vi "HandleFeedForward.vi"(8 "timed out":bool, 11 "Value":u64) -> ()   [LabVIEW 2018]
uses:
  <vilib>/rvi/Memory/Memory_Emulation/nirvimemoryFastEmulation.vi
  <vilib>/rvi/Memory/Memory_Emulation/nirvimemoryEmulation.vi
  <vilib>/rvi/Emulation/niFpgaEmulationIsFPGAContextNoSignature.vi
  <vilib>/rvi/DataTransferAndStorage/Container/Common/niFpgaContainerGetUniqueNameForEmu.vi
  <vilib>/rvi/Emulation/niFpgaProcessEmulError.vi
  <vilib>/rvi/Emulation/niFpgaSctlEmulationGetInTimedLoop.vi
  <vilib>/rvi/errors/nirviReportUnexpectedCaseInternalError (U32).vi
  <vilib>/rvi/FXPMathLib/FxpInterpret/XNode/nifxpmath_Interpret.xnode
  <vilib>/rvi/DataTransferAndStorage/Container/XNode/niFpgaContainer.xnode
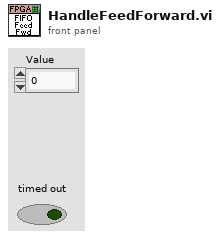
[diagram p1: front panel]
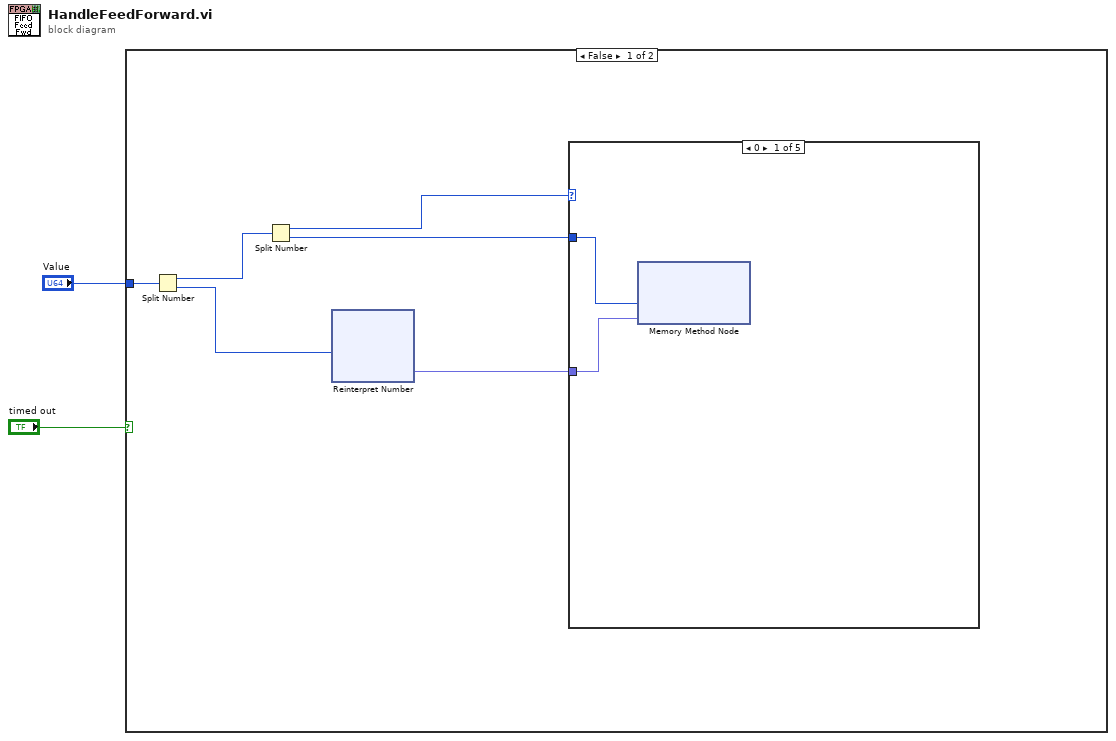
[diagram p0: block diagram]
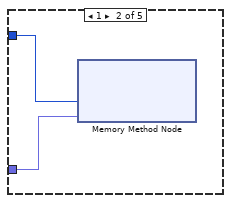
[diagram p2: hidden frame]
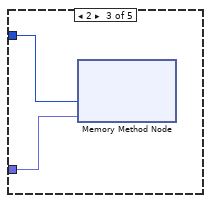
[diagram p3: hidden frame]
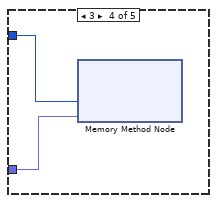
[diagram p4: hidden frame]
diagram:
  n1 = case shown="False" "timed out" {
    tunnel: "Value" -> [w8 _]
    frame False {
      n2 = Split Number(x=w8) -> (hi(x)=w5:u32, lo(x)=w6:u32)
      n3 = Split Number(x=w5) -> (hi(x)=w4:u16, lo(x)=w3:u16)
      n4 = xnode "Reinterpret Number"("x"=w6) -> ("y"=w7:fxp<+/-,32,14>)
      n5 = case shown="0" w4 {
        tunnel: w7 -> [w10 w12 w14 w16 _]
        tunnel: w3 -> [w9 w11 w13 w15 _]
        frame 0 {
          n6 = xnode ("Memory Method Node")("Address"=w9, "Data"=w10) -> ()  [unwired: 1 in, 1 out]
        }
        frame 1 {
          n7 = xnode ("Memory Method Node")("Address"=w11, "Data"=w12) -> ()  [unwired: 1 in, 1 out]
        }
        frame 2 {
          n8 = xnode ("Memory Method Node")("Address"=w13, "Data"=w14) -> ()  [unwired: 1 in, 1 out]
        }
        frame 3 {
          n9 = xnode ("Memory Method Node")("Address"=w15, "Data"=w16) -> ()  [unwired: 1 in, 1 out]
        }
        frame Default {
        }
      }
    }
    frame True {
    }
  }
